vi "test - Cluster mixed with Array 2.vi"(8 "error in (no error)":errorcluster, 11 "TestCase in":refnum<class "testcase-Supported-Datatype.lvclass">) -> (0 "error out":errorcluster, 3 "TestCase out":refnum<class "testcase-Supported-Datatype.lvclass">)   [LabVIEW 2017, in "testcase-Supported-Datatype.lvclass"]
uses:
  testcase-Supported-Datatype.lvclass
  <vilib>/addons/_JKI Toolkits/VI Tester/TestCase.llb/TestCase.lvclass
  addons/API-String-Arugments-Support/API String Arguments Support.lvlib
  C:/Program Files (x86)/National Instruments/LabVIEW 2017/vi.lib/addons/_JKI Toolkits/VI Tester/TestCase.llb/TestCase.lvclass
panel:
  out "Data 3":variant
  out "Data 2":variant
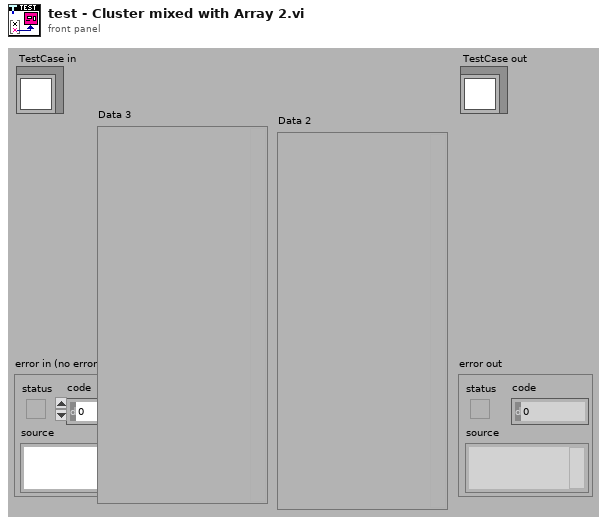
[diagram p1: front panel]
types:
  T1 = cluster{"String":string, "Numberic":i32, "Boolean":bool, "1D Array":dbl[], "2D Array":dbl[][], "Cluster":cluster{"String":string, "Numberic":i32, "Boolean":bool, "1D Array":dbl[], "2D Array":dbl[][]}}
  T2 = cluster{"String":string, "Numberic":i32, "Boolean":bool, "1D Array":dbl[], "2D Array":dbl[][]}
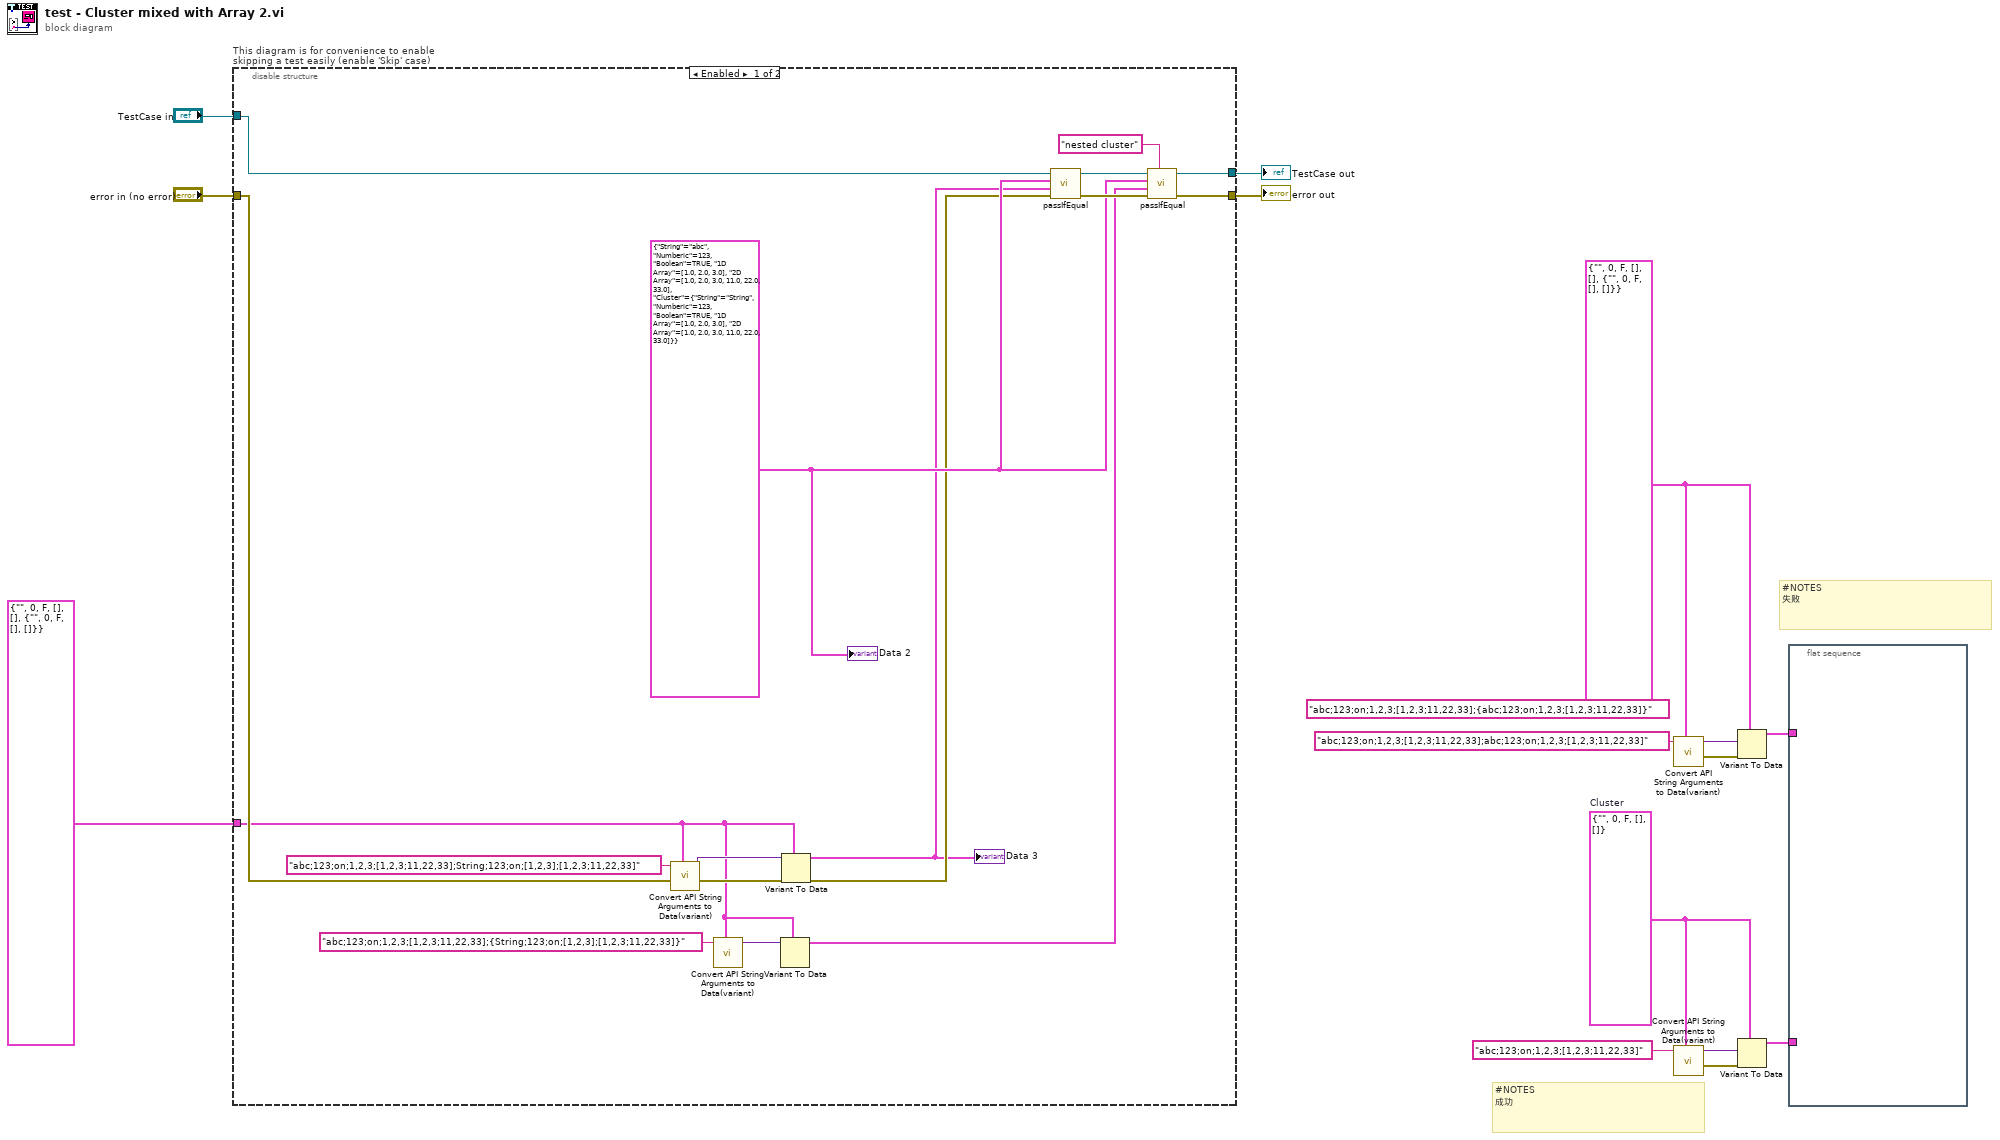
[diagram p0: block diagram]
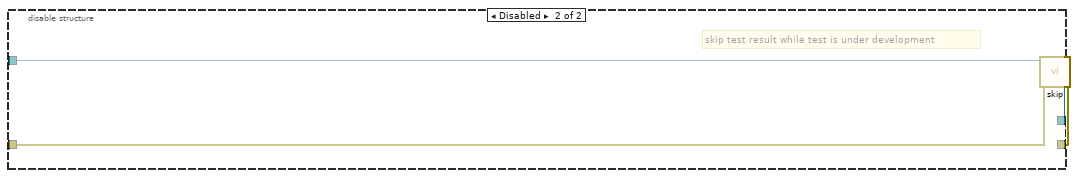
[diagram p2: hidden frame]
diagram:
  (unwired) "abc;123;on;1,2,3;[1,2,3;11,22,33];{abc;123;on;1,2,3;[1,2,3;11,22,33]}" ("String")
  w4 = T1 {"String"="", "Numberic"=0, "Boolean"=FALSE, "1D Array"=[], "2D Array"=[], "Cluster"={"String"="", "Numberic"=0, "Boolean"=FALSE, "1D Array"=[], "2D Array"=[]}}
  w7 = T2 {"String"="", "Numberic"=0, "Boolean"=FALSE, "1D Array"=[], "2D Array"=[]}  # Cluster
  # "#NOTES\n成功"
  # "#NOTES\n失败"
  n1 = disable-structure "This diagram is for convenience to enable skipping a test easily (enable 'Skip' case)" shown="Enabled" {
    disable-tunnel: "TestCase in" -> [w32 w36]
    disable-tunnel: [w26 w34] -> w12
    disable-tunnel: [w25 w35] -> w14
    disable-tunnel: "error in (no error)" -> [w29 w33]
    disable-tunnel: T1 {"String"="", "Numberic"=0, "Boolean"=FALSE, "1D Array"=[], "2D Array"=[], "Cluster"={"String"="", "Numberic"=0, "Boolean"=FALSE, "1D Array"=[], "2D Array"=[]}} -> [w17 _]
    frame Enabled {
      w23 = T1 {"String"="abc", "Numberic"=123, "Boolean"=TRUE, "1D Array"=[1.0, 2.0, 3.0], "2D Array"=[[1.0, 2.0, 3.0], [11.0, 22.0, 33.0]], "Cluster"={"String"="String", "Numberic"=123, "Boolean"=TRUE, "1D Array"=[1.0, 2.0, 3.0], "2D Array"=[[1.0, 2.0, 3.0], [11.0, 22.0, 33.0]]}}
      n2 = call "Convert API String Arguments to Data(variant).vi"("Type"=w17, "error in (no error)"=w29, "String"="abc;123;on;1,2,3;[1,2,3;11,22,33];String;123;on;[1,2,3];[1,2,3;11,22,33]") -> ("error"=w31:errorcluster, "Data"=w20:variant)  [unwired: 7 in]
      n3 = call "Convert API String Arguments to Data(variant).vi"("Type"=w17, "String"="abc;123;on;1,2,3;[1,2,3;11,22,33];{String;123;on;[1,2,3];[1,2,3;11,22,33]}") -> ("Data"=w18:variant)  [unwired: 8 in, 1 out]
      n4 = Variant To Data(type=w17, Variant=w18) -> (data=w16:T1)  [unwired: 1 in, 1 out]
      n5 = Variant To Data(error in=w31, type=w17, Variant=w20) -> (data=w19:T1, error out=w21:errorcluster)
      "Data 3" <- w19
      n6 = call-dynamic "passIfEqual.vi"("error in (no error)"=w21, "y"=w19, "x"=w23, "TestCase in"=w32) -> ("error out"=w24:errorcluster, "TestCase out"=w27:refnum<class "testcase-Supported-Datatype.lvclass">)  [unwired: 6 in]
      n7 = call-dynamic "passIfEqual.vi"("custom report message (\"\")"="nested cluster" ("custom report message (\"\")"), "error in (no error)"=w24, "y"=w16, "x"=w23, "TestCase in"=w27) -> ("error out"=w25:errorcluster, "TestCase out"=w26:refnum<class "testcase-Supported-Datatype.lvclass">)  [unwired: 5 in]
      "Data 2" <- w23
    }
    frame Disabled {
      # "skip test result while test is under development"
      n8 = call <vilib>:"skip.vi"("error in (no error)"=w33, "TestCase in"=w36) -> ("error out"=w35:errorcluster, "TestCase out"=w34:refnum<class "testcase-Supported-Datatype.lvclass">)  [unwired: 8 in]
    }
  }
  "error out" <- w14
  "TestCase out" <- w12
  n9 = call "Convert API String Arguments to Data(variant).vi"("Type"=w4, "String"="abc;123;on;1,2,3;[1,2,3;11,22,33];abc;123;on;1,2,3;[1,2,3;11,22,33]") -> ("error"=w6:errorcluster, "Data"=w5:variant)  [unwired: 8 in]
  n10 = call "Convert API String Arguments to Data(variant).vi"("Type"=w7, "String"="abc;123;on;1,2,3;[1,2,3;11,22,33]") -> ("error"=w9:errorcluster, "Data"=w10:variant)  [unwired: 8 in]
  n11 = Variant To Data(error in=w6, type=w4, Variant=w5) -> (data=w2:T1)  [unwired: 1 out]
  n12 = Variant To Data(error in=w9, type=w7, Variant=w10) -> (data=w1:T2)  [unwired: 1 out]
  n13 = flat-sequence {
    tunnel: w2 -> [_]
    tunnel: w1 -> [_]
    frame #0 {
    }
  }
